vi "Front Switch to Line.vi"(8 "Command Info In":T1, 10 "F-SW--Line":T5, 11 "Starting Position":T4) -> (0 "Command Info Out":T1)   [LabVIEW 2017]
uses:
  Block Clusters/Front Switch to Line.ctl
  Support Code/Starting Position.ctl
  <vilib>/Rock Robotics/WPI/Framework/Command Status Info.ctl
  <vilib>/Rock Robotics/WPI/Framework/Completion Status.ctl
  <vilib>/Rock Robotics/WPI/Framework/Completion Notifier.ctl
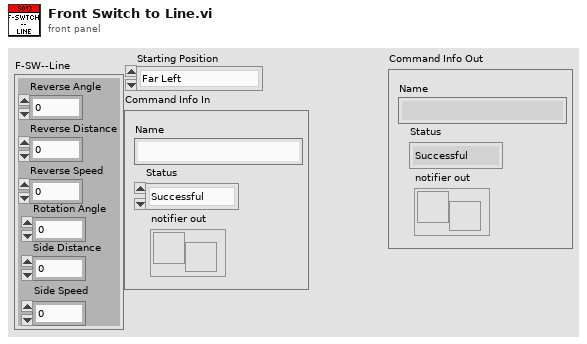
[diagram p1: front panel]
types:
  T1 = typedef "Command Status Info.ctl" = cluster{"Name":string, "Status":T2, "notifier out":T3}
  T2 = typedef "Completion Status.ctl" = enum16{"Successful", "Aborted", "Incomplete"}
  T3 = typedef "Completion Notifier.ctl" = refnum<notifier>
  T4 = typedef "Starting Position.ctl" = enum16{"Far Left", "Center", "Far Right"}
  T5 = typedef "Front Switch to Line.ctl" = cluster{"Reverse Angle":dbl, "Reverse Distance":dbl, "Reverse Speed":dbl, "Rotation Angle":dbl, "Side Distance":dbl, "Side Speed ":dbl}
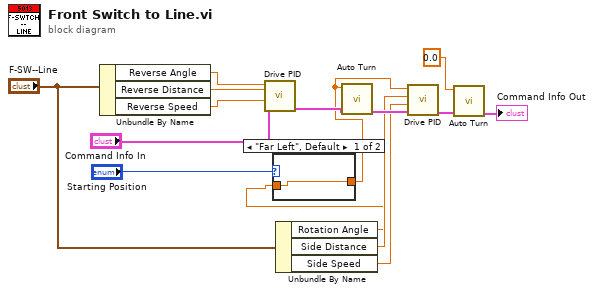
[diagram p0: block diagram]
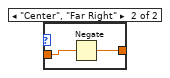
[diagram p2: hidden frame]
diagram:
  n1 = Unbundle By Name("F-SW--Line") -> ("Reverse Angle"=w1:dbl, "Reverse Distance"=w15:dbl, "Reverse Speed"=w14:dbl)
  n2 = call "Drive PID.vi"("Command Info In"="Command Info In", "Speed"=w14, "Distance"=w15, "Target Angle"=w1) -> ("Command Info Out"=w12:T1)  [unwired: 7 in]
  n3 = Unbundle By Name("F-SW--Line") -> ("Rotation Angle"=w3:dbl, "Side Distance"=w9:dbl, "Side Speed"=w8:dbl)
  n4 = case shown="\"Far Left\", Default" "Starting Position" {
    tunnel: w3 -> [w16 w18]
    tunnel: [w16 w17] -> w2
    frame "Far Left", Default {
    }
    frame "Center", "Far Right" {
      n5 = Negate(x=w18) -> (-x=w17:dbl)
    }
  }
  n6 = call "Auto Turn.vi"("Command Info In"=w12, "Target Angle"=w2) -> ("Command Info Out"=w11:T1)  [unwired: 9 in]
  n7 = call "Drive PID.vi"("Command Info In"=w11, "Speed"=w8, "Distance"=w9, "Target Angle"=w2) -> ("Command Info Out"=w7:T1)  [unwired: 7 in]
  n8 = call "Auto Turn.vi"("Command Info In"=w7, "Target Angle"=0.0) -> ("Command Info Out"=→"Command Info Out":T1)  [unwired: 9 in]
